vi "ReadALLColour.vi"(8 "error in (no error)":errorcluster caption="错误输入（无错误）", 11 "CH1603":refnum<visa-resource-name>) -> (1 "数组":i32[](array[numeric]), 2 "布尔":bool, 5 "字符串":string)   [LabVIEW 2015]
uses:
  <vilib>/Instr/_visa.llb/VISA Configure Serial Port (Instr).vi
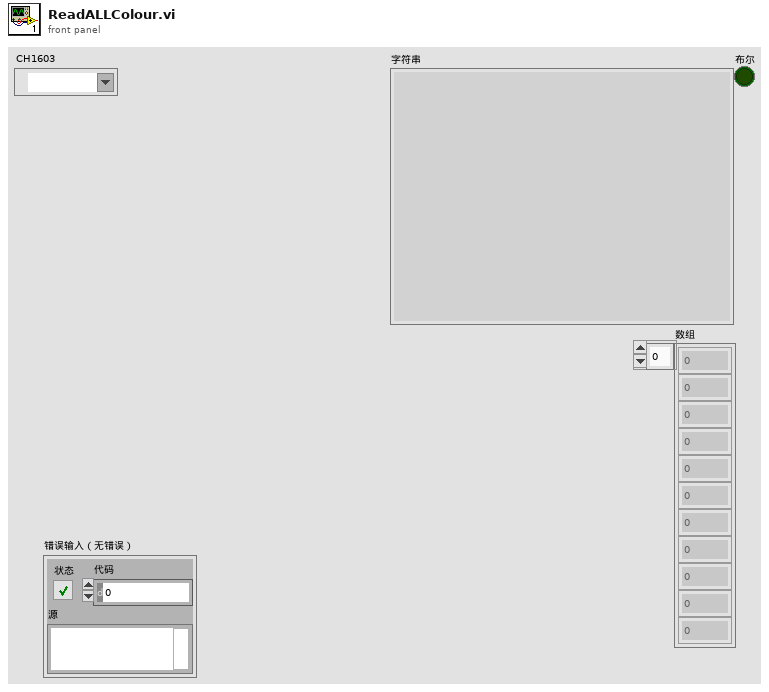
[diagram p1: front panel]
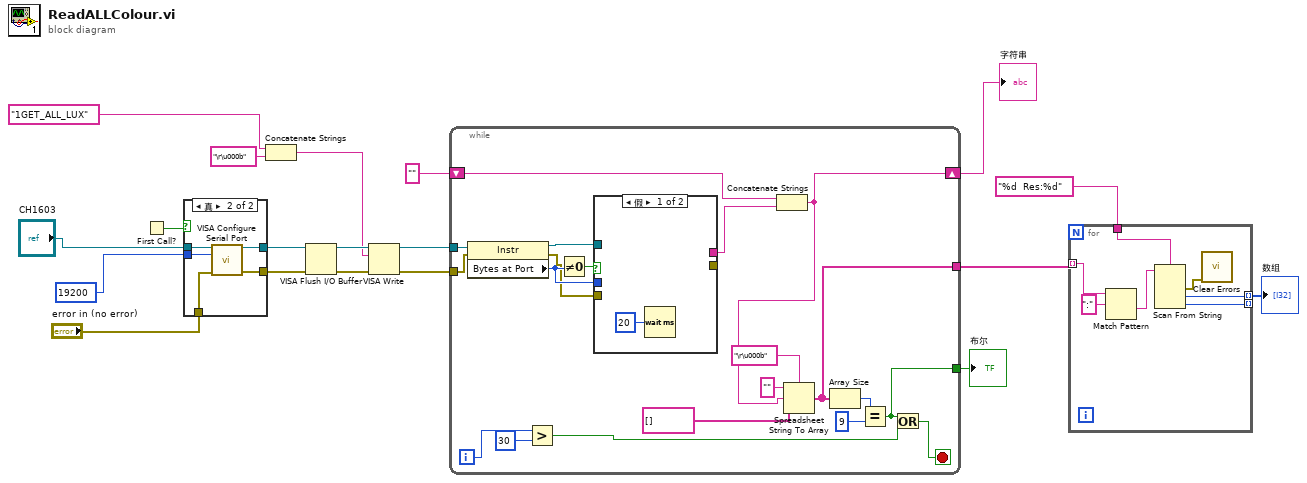
[diagram p0: block diagram]
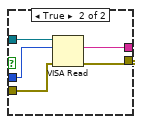
[diagram p2: hidden frame]
diagram:
  n1 = First Call?() -> (First Call?: T/F=w18:bool)
  n2 = case shown="真" w18 {
    tunnel: "error in (no error)" -> [w20 w26]
    tunnel: [w20 w25] -> w11
    tunnel: "CH1603" -> [w21 w24]
    tunnel: [w21 w23] -> w15
    tunnel: u32 19200 ("baud rate (9600)") -> [_ w22]
    frame False {
    }
    frame True {
      n3 = call-poly "VISA Configure Serial Port"("VISA resource name"=w24, "baud rate (9600)"=w22, "error in (no error)"=w26) -> ("VISA resource name out"=w23:refnum<visa-resource-name>, "error out"=w25:errorcluster)  [unwired: 11 in]
    }
  }
  n4 = Concatenate Strings("1GET_ALL_LUX", "\r\u000b" ("字符串")) -> (w10:string)
  n5 = VISA Flush I/O Buffer(VISA resource name=w15, error in (no error)=w11) -> (VISA resource name out=w13:refnum<visa-resource-name>, error out=w12:errorcluster)  [unwired: 1 in]
  n6 = VISA Write(VISA resource name=w13, write buffer=w10, error in (no error)=w12) -> (VISA resource name out=w14:refnum<visa-resource-name>, error out=w9:errorcluster)  [unwired: 1 out]
  n7 = while {
    tunnel: w14 -> [w46]
    tunnel: w9 -> [w44]
    shift-right: [w36] -> w7
    shift-left: "" -> [w40]
    tunnel: [w28] -> w6
    tunnel: [w27] -> w5
    i -> [w32]
    stop <- w29 stop-if-true
    n8 = property class="Instr"(reference=w46, error in=w44) -> (reference out=w43:refnum<visa-resource-name>, error out=w41:errorcluster, "Bytes at Port"=w42:u32)
    n9 = Greater?(x=w32, y=30) -> (0:w30:bool)
    n10 = Not Equal To 0?(x=w42) -> (x != 0?=w45:bool)
    n11 = case shown="假" w45 {
      tunnel: w43 -> [_ w52]
      tunnel: w42 -> [_ w51]
      tunnel: w41 -> [_ w50]
      tunnel: [_ w49] -> _
      tunnel: [_ w48] -> w39
      frame False {
        n12 = Wait (ms)(milliseconds to wait=u32 20 ("等待时间（毫秒）")) -> ()  [unwired: 1 out]
      }
      frame True {
        n13 = VISA Read(VISA resource name=w52, byte count=w51, error in (no error)=w50) -> (read buffer=w48:string, error out=w49:errorcluster)  [unwired: 2 out]
      }
    }
    n14 = Concatenate Strings(w40, w39) -> (w36:string)
    n15 = Spreadsheet String To Array(delimiter (Tab)="\r\u000b" ("分隔符(Tab)"), format string="" ("格式字符串"), spreadsheet string=w36, array type (2D Dbl)=string[] [] ("数组类型(2D Dbl)")) -> (array=w27:string[])
    n16 = Array Size(array=w27) -> (size(s)=w34:i32)
    n17 = Equal?(x=w34, y=9) -> (x = y?=w28:bool)
    n18 = Or(x=w28, y=w30) -> (x .or. y?=w29:bool)
  }
  "字符串" <- w7
  "布尔" <- w6
  n19 = for {
    tunnel: w5 -> [w57] mode=indexing
    tunnel: "%d  Res:%d" ("格式字符串") -> [w59]
    tunnel: [w54] -> w3 mode=indexing
    tunnel: [w53] -> _ mode=indexing
    n20 = Match Pattern(string=w57, regular expression=":" ("正则表达式")) -> (after substring=w58:string)  [unwired: 1 in, 3 out]
    n21 = Scan From String(format string=w59, input string=w58) -> (error out=w55:errorcluster, output 1=w54:i32, output 2=w53:i32)  [unwired: 4 in, 2 out]
    n22 = call <vilib>:"Clear Errors.vi"("error in (no error)"=w55) -> ()  [unwired: 5 in, 2 out]
  }
  "数组" <- w3
